vi "Voltage - SW-Timed Input-Jitter.vi"() -> ()   [LabVIEW 2014]
doc: "This example demonstrates how to acquire data based off of software timing.\n\nFor instructions on how to connect your signals to the DAQ device, refer to your device documentation."
uses:
  <vilib>/Utility/error.llb/DialogType.ctl
  <vilib>/DAQmx/create/channels.llb/DAQmx Create Channel (AI-Voltage-Basic).vi
  <vilib>/DAQmx/read.llb/DAQmx Read (Analog Wfm 1Chan 1Samp).vi
panel:
  out "Sample Rate (Hz)":dbl=100.0 format="%#.3p"
  out "Jitter":waveform(dbl)(graph)
  in  "Loop Time (ms)":i32=100
  in  "Stop":bool
  out "Waveform Chart":waveform(dbl)(graph)
  in  "Terminal Configuration":i32(ring)=-1 items=["default"=-1, "RSE"=10083, "NRSE"=10078, "Differential"=10106, "Pseudodifferential"=12529]
  in  "Max Voltage":dbl=5.0
  in  "Min Voltage":dbl=-5.0
  in  "Physical Channel":tag="Dev1/ai0"
  # "Channel Settings"
  # "Acquired Data"
  # "Timing Settings"
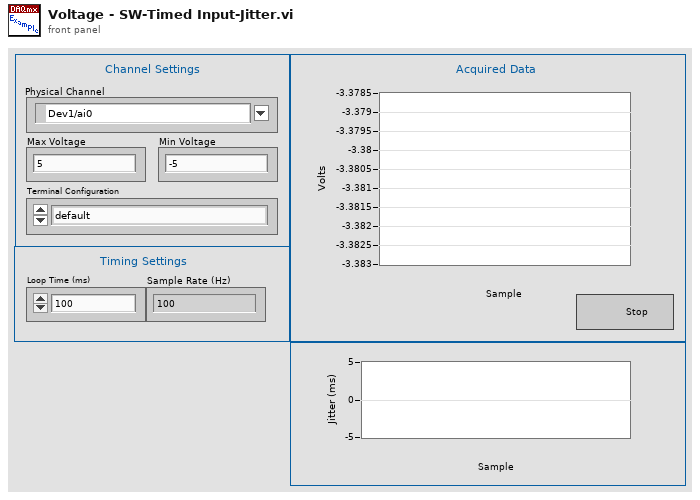
[diagram p1: front panel]
types:
  T1 = typedef "DialogType.ctl" = u16
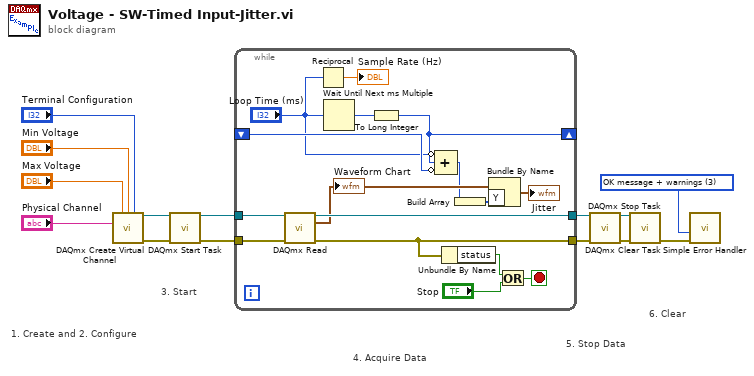
[diagram p0: block diagram]
diagram:
  w1 = T1 3 items=["no dialog", "OK message", "continue or stop message", "OK message + warnings", "continue/stop + warnings"] ("type of dialog (OK msg:1)")
  # "6. Clear"
  # "5. Stop Data"
  # "3. Start"
  # "4. Acquire Data"
  # "1. Create and 2. Configure"
  n1 = call-poly <vilib>:"DAQmx Create Virtual Channel.vi"("maximum value"="Max Voltage", "minimum value"="Min Voltage", "input terminal configuration"="Terminal Configuration", "physical channels"="Physical Channel") -> ("task out"=w6:refnum<k21>, "error out"=w7:errorcluster)  [unwired: 10 in]
  n2 = call <vilib>:"DAQmx Start Task.vi"("task/channels in"=w6, "error in"=w7) -> ("task out"=w14:refnum<k21>, "error out"=w13:errorcluster)  [unwired: 12 in]
  n3 = while {
    tunnel: w14 -> [w30]
    tunnel: w13 -> [w29]
    tunnel: [w26] -> w2
    tunnel: [w27] -> w3
    shift-right: [w17] -> _
    shift-left: _ -> [w22]
    stop <- w28 stop-if-true
    n4 = call-poly <vilib>:"DAQmx Read.vi"("task/channels in"=w30, "error in"=w29) -> ("task out"=w27:refnum<k21>, "data"=w21:waveform(dbl), "error out"=w26:errorcluster)  [unwired: 11 in]
    "Waveform Chart" <- w21
    n5 = Reciprocal(x="Loop Time (ms)") -> (1/x=→"Sample Rate (Hz)":dbl)
    n6 = Wait Until Next ms Multiple(millisecond multiple="Loop Time (ms)") -> (millisecond timer value=w23:u32)
    n7 = To Long Integer(number=w23) -> (32bit integer=w17:i32)
    n8 = Compound Arithmetic op=ADD(invert "Loop Time (ms)", w17, invert w22) -> (w20:i32)
    n9 = Unbundle By Name(w26) -> ("status"=w25:bool)
    n10 = Build Array(w20) -> (w19:i32[])
    n11 = Bundle By Name(cluster=w21, "Y"=w19) -> (→"Jitter":waveform(dbl))
    n12 = Or(x=w25, y="Stop") -> (x .or. y?=w28:bool)
  }
  n13 = call <vilib>:"DAQmx Stop Task.vi"("task/channels in"=w3, "error in"=w2) -> ("task out"=w5:refnum<k21>, "error out"=w4:errorcluster)  [unwired: 12 in]
  n14 = call <vilib>:"DAQmx Clear Task.vi"("task in"=w5, "error in"=w4) -> ("error out"=w12:errorcluster)  [unwired: 13 in]
  n15 = call <vilib>:"Simple Error Handler.vi"("type of dialog (OK msg:1)"=w1, "error in (no error)"=w12) -> ()  [unwired: 3 in, 5 out]
